vi "APP Close Stand Alone Interface.vi"(1 "APP Setup In":T1, 2 "Display Ref":refnum<vi>, 11 "Error In (no error)":errorcluster, 12 "Stand Alone (F)":bool) -> (15 "Error Out":errorcluster)   [LabVIEW 2011]
uses:
  Type Defs/APP Application Setup Cluster.ctl
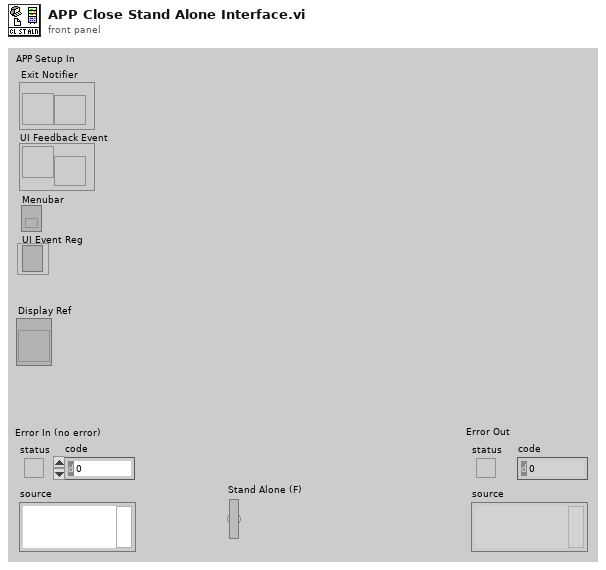
[diagram p1: front panel]
types:
  T1 = typedef "APP Application Setup Cluster.ctl" = cluster{"Menubar":refnum<k9>, "Exit Notifier":refnum<notifier>, "UI Feedback Event":refnum<user-event>, "UI Event Reg":refnum<event-registration>}
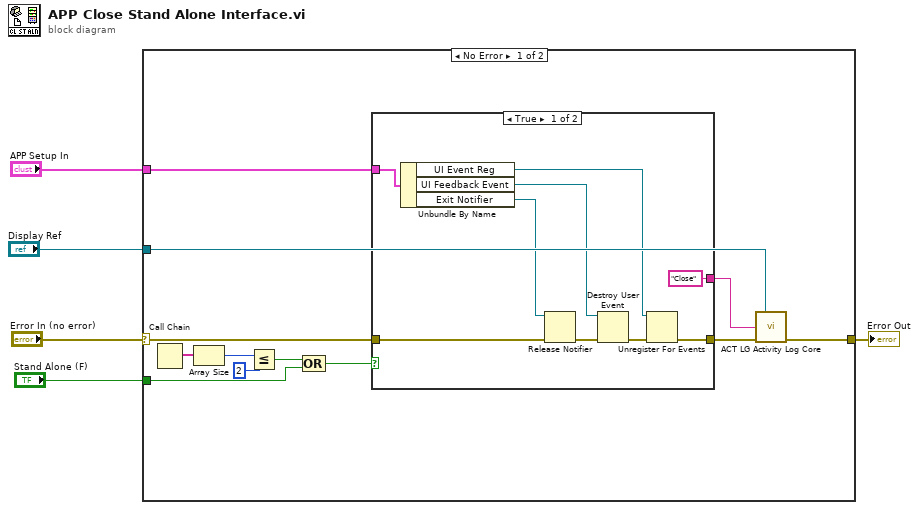
[diagram p0: block diagram]
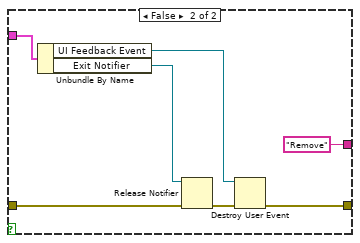
[diagram p2: hidden frame]
diagram:
  n1 = case shown="No Error" "Error In (no error)" {
    selector: "Error In (no error)" -> [w15 w34]
    tunnel: [w13 w34] -> w5
    tunnel: "APP Setup In" -> [w17 _]
    tunnel: "Display Ref" -> [w12 _]
    tunnel: "Stand Alone (F)" -> [w8 _]
    frame No Error {
      n2 = Call Chain() -> (call chain=w16:string[])
      n3 = Array Size(array=w16) -> (size(s)=w10:i32)
      n4 = Less Or Equal?(x=w10, y=2) -> (x <= y?=w7:bool)
      n5 = Compound Arithmetic op=OR(w7, w8) -> (w6:bool)
      n6 = case shown="True" w6 {
        tunnel: w15 -> [w26 w33]
        tunnel: [w20 w28] -> w14
        tunnel: w17 -> [w24 w31]
        tunnel: ["Close" ("Log Line") "Remove" ("Log Line")] -> w11
        frame True {
          n7 = Unbundle By Name(w24) -> ("UI Event Reg"=w19:refnum<event-registration>, "UI Feedback Event"=w23:refnum<user-event>, "Exit Notifier"=w22:refnum<notifier>)
          n8 = Release Notifier(notifier=w22, error in (no error)=w26) -> (error out=w25:errorcluster)  [unwired: 3 out]
          n9 = Destroy User Event(user event=w23, error in=w25) -> (error out=w21:errorcluster)
          n10 = Unregister For Events(event registration refnum=w19, error in=w21) -> (error out=w20:errorcluster)
        }
        frame False {
          n11 = Unbundle By Name(w31) -> ("UI Feedback Event"=w30:refnum<user-event>, "Exit Notifier"=w29:refnum<notifier>)
          n12 = Release Notifier(notifier=w29, error in (no error)=w33) -> (error out=w32:errorcluster)  [unwired: 3 out]
          n13 = Destroy User Event(user event=w30, error in=w32) -> (error out=w28:errorcluster)
        }
      }
      n14 = call "ACT LG Activity Log Core.vi"("Display Ref"=w12, "Log Line"=w11, "Error In (no error)"=w14) -> ("Error Out"=w13:errorcluster)  [unwired: 2 in, 10 out]
    }
    frame Error {
    }
  }
  "Error Out" <- w5
